vi "test PLC.vi"() -> ()   [LabVIEW 2017]
uses:
  <vilib>/NI/Modbus Library/API/Wrapper/Create TCP Master.vi
  <vilib>/NI/Modbus Library/API/master/Modbus Master.lvclass
  <vilib>/NI/Modbus Library/API/Wrapper/API Main.lvlib
  <vilib>/ptbypt/NI_PtbyPt.lvlib
panel:
  out "status":bool
  out "Boolean array":bool[](array[boolean])
  out "crossing count":i32
  out "gate count":i32
  in  "stop":bool
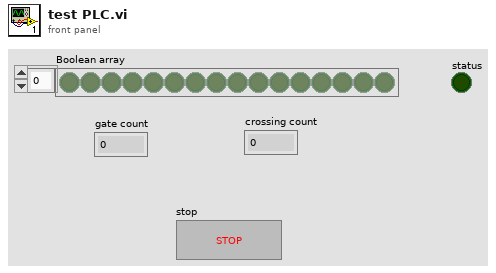
[diagram p1: front panel]
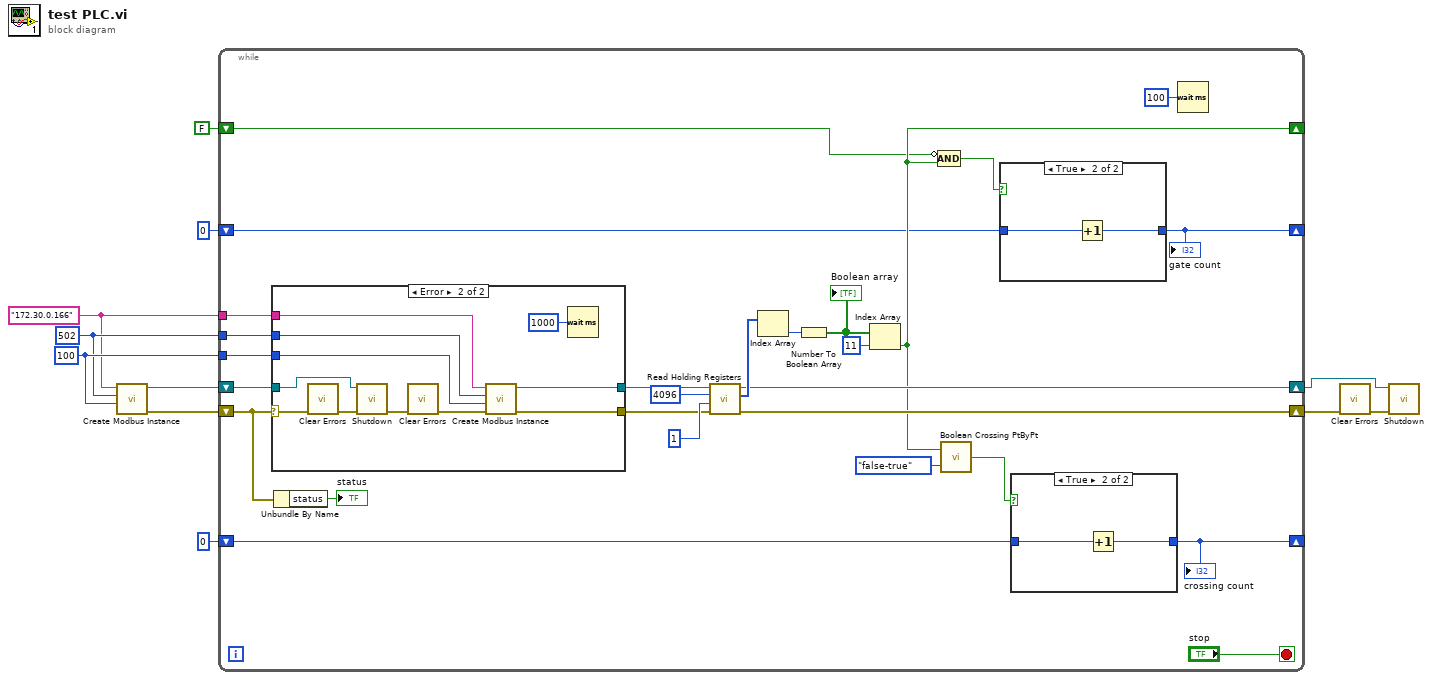
[diagram p0: block diagram]
diagram:
  w7 = "172.30.0.166" ("address")
  w8 = u16 502 ("port (502)")
  w9 = 100 ("connect timeout ms")
  n1 = call-poly <vilib>:"Create Modbus Instance.vi"("connect timeout ms"=w9, "port (502)"=w8, "address"=w7) -> ("error out"=w10:errorcluster, "TCP master instance"=w11:refnum<class "Modbus Master.lvclass">)  [unwired: 7 in]
  n2 = while {
    tunnel: w9 -> [w37]
    tunnel: w8 -> [w36]
    tunnel: w7 -> [w35]
    shift-right: [w24] -> w1
    shift-left: w11 -> [w38]
    shift-right: [w23] -> w2
    shift-left: w10 -> [w13]
    shift-right: [w21] -> _
    shift-left: FALSE -> [w20]
    shift-right: [w18] -> _
    shift-left: 0 -> [w17]
    shift-right: [w15] -> _
    shift-left: 0 -> [w14]
    stop <- "stop" stop-if-true
    n3 = case shown="Error" w13 {
      selector: w13 -> [w45 w51]
      tunnel: w38 -> [w46 w50]
      tunnel: [w46 w55] -> w30
      tunnel: [w45 w54] -> w29
      tunnel: w35 -> [_ w47]
      tunnel: w36 -> [_ w48]
      tunnel: w37 -> [_ w49]
      frame No Error {
      }
      frame Error {
        n4 = call <vilib>:"Clear Errors.vi"("error in (no error)"=w51) -> ("error out"=w53:errorcluster)  [unwired: 5 in, 1 out]
        n5 = call-dynamic "Shutdown.vi"("error in"=w53, "Modbus master in"=w50) -> ("error out"=w57:errorcluster)  [unwired: 9 in]
        n6 = call <vilib>:"Clear Errors.vi"("error in (no error)"=w57) -> ("error out"=w56:errorcluster)  [unwired: 5 in, 1 out]
        n7 = call-poly <vilib>:"Create Modbus Instance.vi"("error in"=w56, "connect timeout ms"=w49, "port (502)"=w48, "address"=w47) -> ("error out"=w54:errorcluster, "TCP master instance"=w55:refnum<class "Modbus Master.lvclass">)  [unwired: 6 in]
        n8 = Wait (ms)(milliseconds to wait=u32 1000) -> ()  [unwired: 1 out]
      }
    }
    n9 = Unbundle By Name(w13) -> ("status"=→"status":bool)
    n10 = call-dynamic "Read Holding Registers.vi"("error in"=w29, "number of inputs"=u16 1, "starting address"=u16 4096, "Modbus master in"=w30) -> ("error out"=w23:errorcluster, "register values"=w28:u16[], "Modbus master out"=w24:refnum<class "Modbus Master.lvclass">)  [unwired: 5 in]
    n11 = Index Array(array=w28) -> (element=w27:u16)  [unwired: 1 in]
    n12 = Number To Boolean Array(number=w27) -> (Boolean array=w26:bool[])
    "Boolean array" <- w26
    n13 = Index Array(array=w26, index=11) -> (element=w21:bool)
    n14 = Compound Arithmetic op=AND(invert w20, w21) -> (w16:bool)
    n15 = call <vilib>:"Boolean Crossing PtByPt.vi"("direction"=enum16{"either", "false-true", "true-false"}."false-true", "input"=w21) -> ("crossing"=w19:bool)  [unwired: 1 in]
    n16 = case shown="True" w16 {
      tunnel: [w39 w41] -> w15
      tunnel: w14 -> [w39 w40]
      frame False {
      }
      frame True {
        n17 = Increment(x=w40) -> (x+1=w41:i32)
      }
    }
    "gate count" <- w15
    n18 = case shown="True" w19 {
      tunnel: [w42 w44] -> w18
      tunnel: w17 -> [w42 w43]
      frame False {
      }
      frame True {
        n19 = Increment(x=w43) -> (x+1=w44:i32)
      }
    }
    "crossing count" <- w18
    n20 = Wait (ms)(milliseconds to wait=u32 100) -> ()  [unwired: 1 out]
  }
  n21 = call <vilib>:"Clear Errors.vi"("error in (no error)"=w2) -> ("error out"=w3:errorcluster)  [unwired: 5 in, 1 out]
  n22 = call-dynamic "Shutdown.vi"("error in"=w3, "Modbus master in"=w1) -> ()  [unwired: 9 in, 1 out]
